vi "EMG - Mean and Median Frequency.vi"() -> ()   [LabVIEW 2013]
uses:
  <vilib>/addons/Biomedical/Biosignal Measurements/EMG/EMG Median Power Frequency (Waveform).vi
  <vilib>/addons/Biomedical/Biosignal Measurements/EMG/EMG Mean Power Frequency (Waveform).vi
  <vilib>/addons/Biomedical/NI_BMTK_Measurements.lvlib
panel:
  in  "Podesavanja prozora":cluster{"tip":i32, "duzina":i32}={"tip"=1, "duzina"=-1} {"tip" items=["None ", "Hanning", "Hamming", "Blackman-Harris", "Exact Blackman", "Blackman", "Flat Top", "4 Term B-Harris ", "7 Term B-Harris", "Low Sidelobe", "Gaussian"]}
  out "Lokacija sacuvanog fajla na racunaru (medijana frekvencija)":path
  out "Snaga medijana frekvencije":cluster{"t0":dbl, "dt":dbl, "frequency":dbl[]}(graph)
  out "Lokacija sacuvanog fajla na racunaru (srednja frekvencija)":path
  out "Snaga srednje frekvencije":cluster{"t0":dbl, "dt":dbl, "frequency":dbl[]}(graph)
  in  "Podesavanja vremena i frekvencije":T1={"vremenski koraci"=-1, "frekventni binovi"=512}
  out "Signal pre analize":waveform(dbl)[](graph)
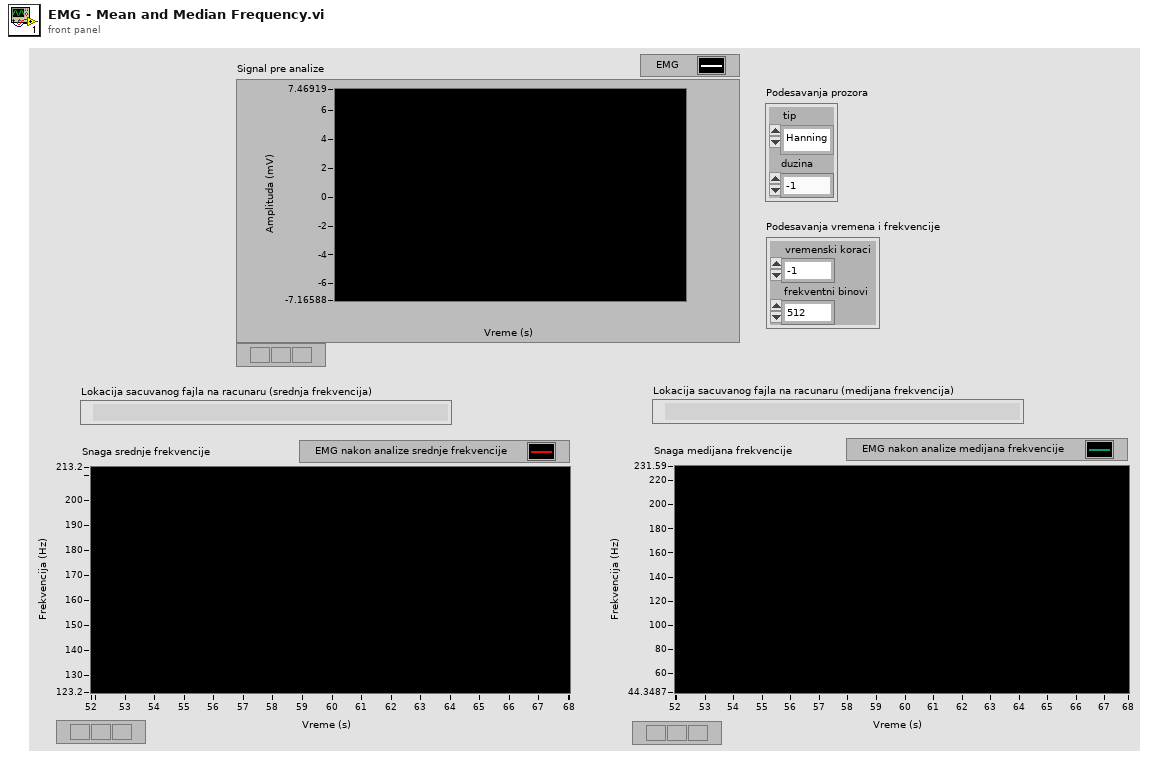
[diagram p1: front panel]
types:
  T1 = cluster{"vremenski koraci":i32, "frekventni binovi":i32}
  T2 = enum16{"open", "open or create", "create or replace", "create", "open (read-only)"}
  T3 = enum16{"open", "replace", "create", "open or create", "replace or create", "replace or create with confirmation"}
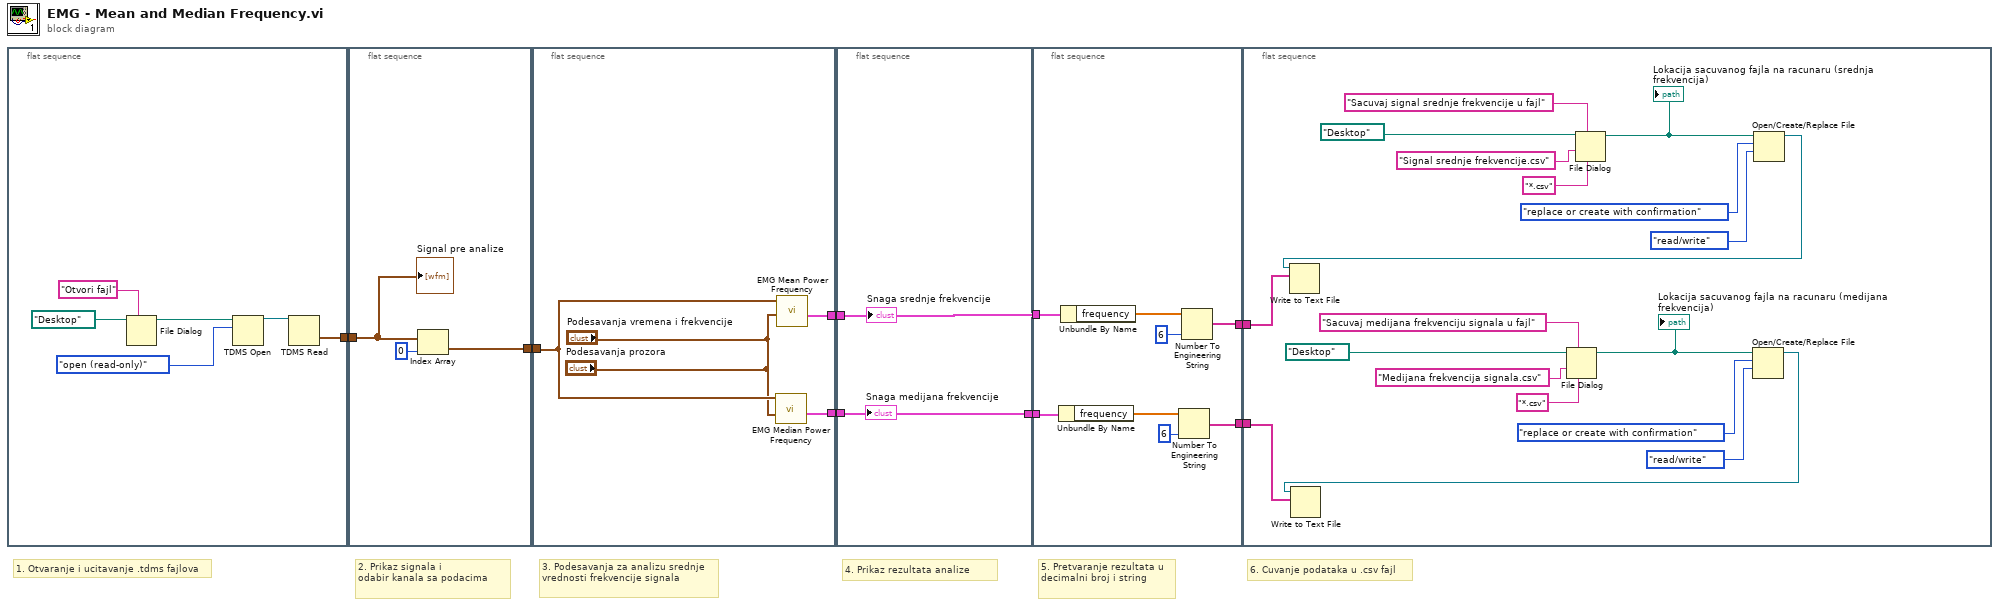
[diagram p0: block diagram]
diagram:
  # "6. Cuvanje podataka u .csv fajl"
  # "5. Pretvaranje rezultata u decimalni broj i string"
  # "4. Prikaz rezultata analize"
  # "3. Podesavanja za analizu srednje vrednosti frekvencije signala"
  # "2. Prikaz signala i \nodabir kanala sa podacima"
  # "1. Otvaranje i ucitavanje .tdms fajlova"
  n1 = flat-sequence {
    tunnel: [w9] -> w7
    frame #0 {
      n2 = File Dialog(7:"Otvori fajl" ("prompt"), 11:path "/Desktop" ("start path")) -> (3:w11:path)  [unwired: 2 in, 6 out]
      n3 = TDMS Open(10:T2."open (read-only)" ("operation (0:open)"), 11:w11) -> (3:w12:refnum<k34>)  [unwired: 5 in, 1 out]
      n4 = TDMS Read(0:w12) -> (10:w9:waveform(dbl)[])  [unwired: 7 in, 5 out]
    }
  }
  n5 = flat-sequence {
    tunnel: w7 -> [w16]
    tunnel: [w14] -> w6
    frame #0 {
      n6 = Index Array(array=w16, index=0) -> (element=w14:waveform(dbl))
      "Signal pre analize" <- w16
    }
  }
  n7 = flat-sequence {
    tunnel: w6 -> [w20]
    tunnel: [w21] -> w4
    tunnel: [w19] -> w3
    frame #0 {
      n8 = call-poly <vilib>:"EMG Median Power Frequency.vi"("window info"="Podesavanja prozora", "time-freq sampling info"="Podesavanja vremena i frekvencije", "EMG"=w20) -> ("MDF"=w19:cluster{"t0":dbl, "dt":dbl, "frequency":dbl[]})  [unwired: 5 in, 3 out]
      n9 = call-poly <vilib>:"EMG Mean Power Frequency.vi"("window info"="Podesavanja prozora", "time-freq sampling info"="Podesavanja vremena i frekvencije", "EMG"=w20) -> ("MNF"=w21:cluster{"t0":dbl, "dt":dbl, "frequency":dbl[]})  [unwired: 5 in, 3 out]
    }
  }
  n10 = flat-sequence {
    tunnel: w4 -> [w23]
    tunnel: w3 -> [w22]
    tunnel: [w22] -> w2
    frame #0 {
      "Snaga srednje frekvencije" <- w23
      "Snaga medijana frekvencije" <- w22
    }
  }
  n11 = flat-sequence {
    tunnel: [w31] -> w5
    tunnel: w4 -> [w29]
    tunnel: w2 -> [w25]
    tunnel: [w24] -> w1
    frame #0 {
      n12 = Unbundle By Name(w25) -> ("frequency"=w26:dbl[])
      n13 = Unbundle By Name(w29) -> ("frequency"=w28:dbl[])
      n14 = Number To Engineering String(2:i16 6 ("precision (6)"), 4:w26) -> (0:w24:string[])  [unwired: 2 in]
      n15 = Number To Engineering String(2:i16 6 ("precision (6)"), 4:w28) -> (0:w31:string[])  [unwired: 2 in]
    }
  }
  n16 = flat-sequence {
    tunnel: w5 -> [w42]
    tunnel: w1 -> [w34]
    frame #0 {
      n17 = File Dialog(6:"*.csv" ("pattern (all files)"), 7:"Sacuvaj medijana frekvenciju signala u fajl" ("prompt"), 9:"Medijana frekvencija signala.csv" ("default name"), 11:path "/Desktop" ("start path")) -> (3:w36:path)  [unwired: 1 in, 5 out]
      "Lokacija sacuvanog fajla na racunaru (medijana frekvencija)" <- w36
      n18 = File Dialog(6:"*.csv" ("pattern (all files)"), 7:"Sacuvaj signal srednje frekvencije u fajl" ("prompt"), 9:"Signal srednje frekvencije.csv" ("default name"), 11:path "/Desktop" ("start path")) -> (3:w44:path)  [unwired: 1 in, 5 out]
      "Lokacija sacuvanog fajla na racunaru (srednja frekvencija)" <- w44
      n19 = Open/Create/Replace File(file path (use dialog)=w36, operation (0:open)=T3."replace or create with confirmation", access (0:read/write)=enum16{"read/write", "read-only", "write-only"}."read/write") -> (refnum out=w33:refnum<file>)  [unwired: 3 in, 2 out]
      n20 = Write to Text File(file (use dialog)=w33, text=w34) -> ()  [unwired: 2 in, 3 out]
      n21 = Open/Create/Replace File(file path (use dialog)=w44, operation (0:open)=T3."replace or create with confirmation", access (0:read/write)=enum16{"read/write", "read-only", "write-only"}."read/write") -> (refnum out=w41:refnum<file>)  [unwired: 3 in, 2 out]
      n22 = Write to Text File(file (use dialog)=w41, text=w42) -> ()  [unwired: 2 in, 3 out]
    }
  }
